vi "FilterHemisphereGPS.vi"(9 "Queue timeout (ms)":i32=200, 10 "NotifierReff":T2, 11 "Hemisphere Queue Cluster":T1) -> ()   [LabVIEW 2013]
doc: "Performs and filtering that we want (default is no filtering) and writes the data to the notifier. If no data is in the queue this VI times out after 'Queue timeout (ms)' has passed and nothing is written to the notifier.\n\nEric Schneider, March 2014"
uses:
  Data/TypeDefs/Notifiers.ctl
  Data/TypeDefs/UTM Location.ctl
  Data/TypeDefs/Sail Set Suggestions.ctl
  Data/TypeDefs/Rudder Set Suggestions.ctl
  Data/TypeDefs/OverrideInformation.ctl
  Data/TypeDefs/OverrideMode.ctl
  Data/TypeDefs/MotorSetup.ctl
  Data/TypeDefs/DynamixelSetupInfo.ctl
  Data/TypeDefs/AirmarStatus.ctl
  Data/TypeDefs/HardwareOnline.ctl
  Data/TypeDefs/DynamixelCycleTracker.ctl
  Data/TypeDefs/RC Input Values.ctl
  Classes/Waypoint/Waypoint.lvclass
  Data/TypeDefs/GPS-Compass Queue Cluster.ctl
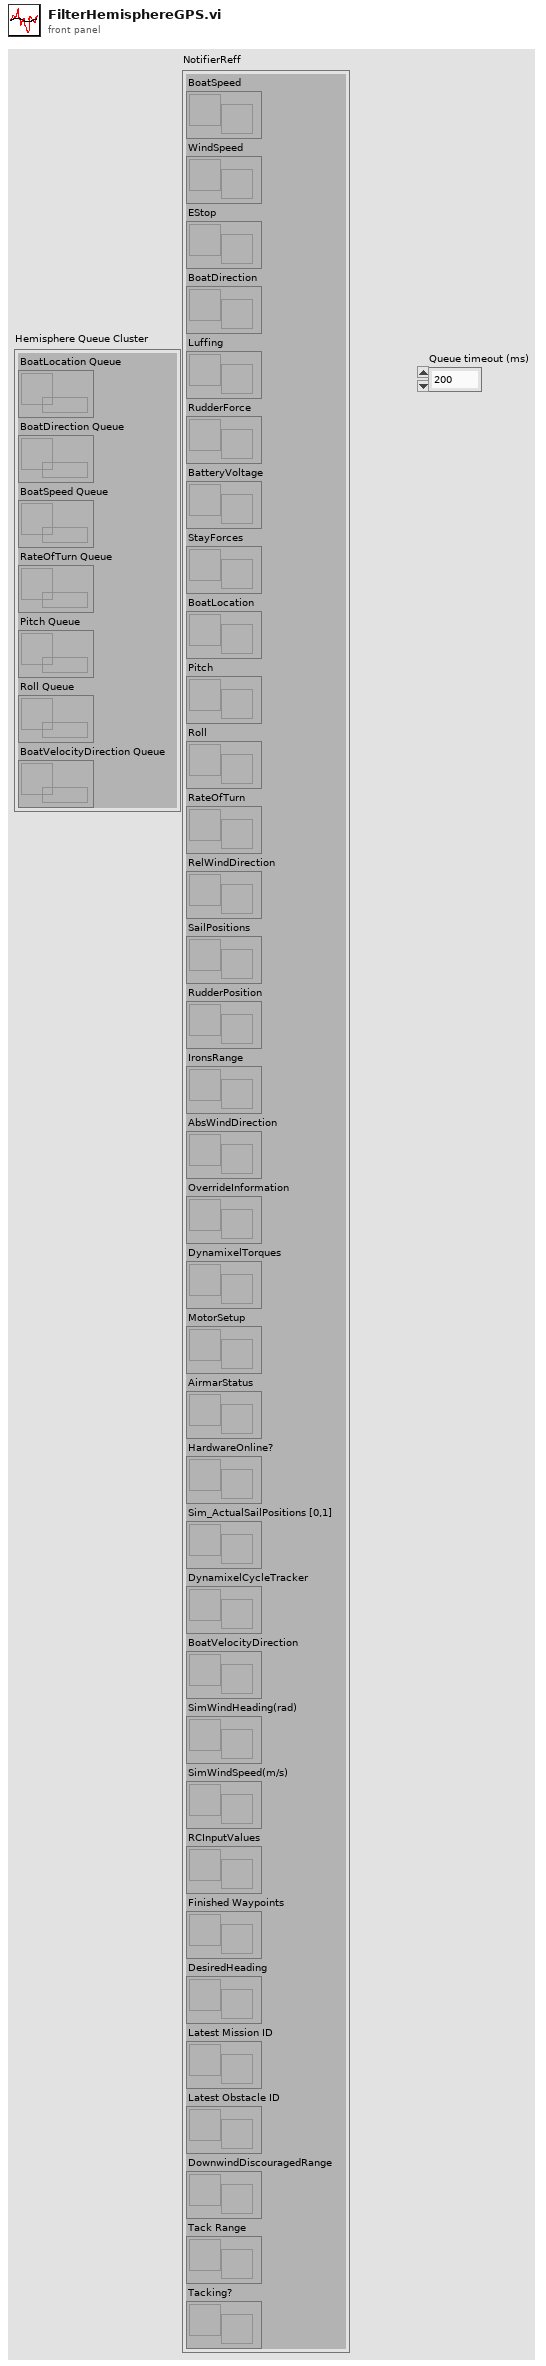
[diagram p1: front panel]
types:
  T1 = typedef "GPS-Compass Queue Cluster.ctl" = cluster{"BoatLocation Queue":refnum<queue>, "BoatDirection Queue":refnum<queue>, "BoatSpeed Queue":refnum<queue>, "RateOfTurn Queue":refnum<queue>, "Pitch Queue":refnum<queue>, "Roll Queue":refnum<queue>, "BoatVelocityDirection Queue ":refnum<queue>}
  T2 = typedef "Notifiers.ctl" = cluster{"BoatSpeed":refnum<notifier>, "WindSpeed":refnum<notifier>, "EStop":refnum<notifier>, "BoatDirection":refnum<notifier>, "Luffing":refnum<notifier>, "RudderForce":refnum<notifier>, "BatteryVoltage":refnum<notifier>, "StayForces":refnum<notifier>, "BoatLocation":refnum<notifier>, "Pitch":refnum<notifier>, "Roll":refnum<notifier>, "RateOfTurn":refnum<notifier>, "RelWindDirection":refnum<notifier>, "SailPositions":refnum<notifier>, "RudderPosition":refnum<notifier>, "IronsRange":refnum<notifier>, "AbsWindDirection":refnum<notifier>, "OverrideInformation":refnum<notifier>, "DynamixelTorques":refnum<notifier>, "MotorSetup":refnum<notifier>, "AirmarStatus":refnum<notifier>, "HardwareOnline?":refnum<notifier>, "Sim_ActualSailPositions [0,1]":refnum<notifier>, "DynamixelCycleTracker":refnum<notifier>, "BoatVelocityDirection":refnum<notifier>, "SimWindHeading(rad)":refnum<notifier>, "SimWindSpeed(m/s)":refnum<notifier>, "RCInputValues":refnum<notifier>, "Finished Waypoints":refnum<notifier>, "DesiredHeading":refnum<notifier>, "Latest Mission ID":refnum<notifier>, "Latest Obstacle ID":refnum<notifier>, "DownwindDiscouragedRange":refnum<notifier>, "Tack Range":refnum<notifier>, "Tacking?":refnum<notifier>}
  T3 = typedef "UTM Location.ctl" = cluster{"UTM Zone":dbl, "Hemisphere":enum16{"North", "South"}, "East":dbl, "North":dbl}
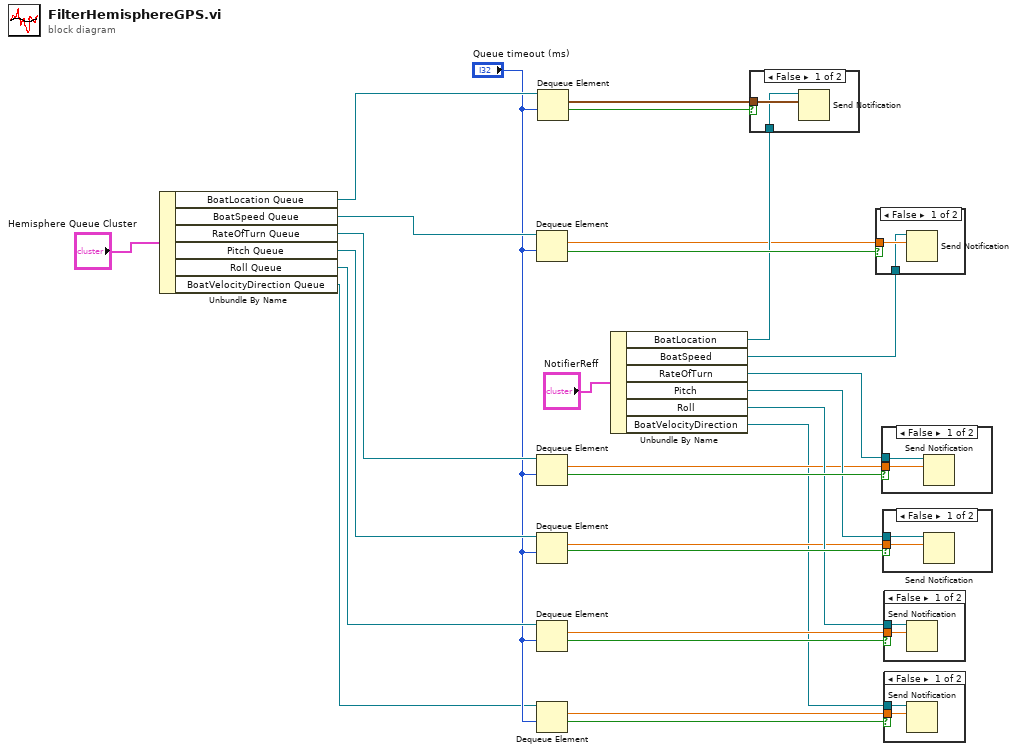
[diagram p0: block diagram]
diagram:
  n1 = Unbundle By Name("Hemisphere Queue Cluster") -> ("BoatLocation Queue"=w7:refnum<queue>, "BoatSpeed Queue"=w8:refnum<queue>, "RateOfTurn Queue"=w9:refnum<queue>, "Pitch Queue"=w10:refnum<queue>, "Roll Queue"=w11:refnum<queue>, "BoatVelocityDirection Queue"=w4:refnum<queue>)
  n2 = Dequeue Element(queue=w8, timeout in ms (-1)="Queue timeout (ms)") -> (element=w14:dbl, timed out?=w24:bool)  [unwired: 1 in, 2 out]
  n3 = Dequeue Element(queue=w9, timeout in ms (-1)="Queue timeout (ms)") -> (element=w13:dbl, timed out?=w25:bool)  [unwired: 1 in, 2 out]
  n4 = Dequeue Element(queue=w10, timeout in ms (-1)="Queue timeout (ms)") -> (element=w15:dbl, timed out?=w26:bool)  [unwired: 1 in, 2 out]
  n5 = Dequeue Element(queue=w11, timeout in ms (-1)="Queue timeout (ms)") -> (element=w16:dbl, timed out?=w27:bool)  [unwired: 1 in, 2 out]
  n6 = Dequeue Element(queue=w4, timeout in ms (-1)="Queue timeout (ms)") -> (element=w2:dbl, timed out?=w3:bool)  [unwired: 1 in, 2 out]
  n7 = Dequeue Element(queue=w7, timeout in ms (-1)="Queue timeout (ms)") -> (element=w12:T3, timed out?=w23:bool)  [unwired: 1 in, 2 out]
  n8 = Unbundle By Name("NotifierReff") -> ("BoatLocation"=w18:refnum<notifier>, "BoatSpeed"=w19:refnum<notifier>, "RateOfTurn"=w20:refnum<notifier>, "Pitch"=w21:refnum<notifier>, "Roll"=w22:refnum<notifier>, "BoatVelocityDirection"=w1:refnum<notifier>)
  n9 = case shown="False" w23 {
    tunnel: w12 -> [w29 _]
    tunnel: w18 -> [w28 _]
    frame False {
      n10 = Send Notification(notification=w29, notifier=w28) -> ()  [unwired: 1 in, 2 out]
    }
    frame True {
    }
  }
  n11 = case shown="False" w24 {
    tunnel: w14 -> [w31 _]
    tunnel: w19 -> [w30 _]
    frame False {
      n12 = Send Notification(notification=w31, notifier=w30) -> ()  [unwired: 1 in, 2 out]
    }
    frame True {
    }
  }
  n13 = case shown="False" w25 {
    tunnel: w13 -> [w33 _]
    tunnel: w20 -> [w32 _]
    frame False {
      n14 = Send Notification(notification=w33, notifier=w32) -> ()  [unwired: 1 in, 2 out]
    }
    frame True {
    }
  }
  n15 = case shown="False" w26 {
    tunnel: w15 -> [w35 _]
    tunnel: w21 -> [w34 _]
    frame False {
      n16 = Send Notification(notification=w35, notifier=w34) -> ()  [unwired: 1 in, 2 out]
    }
    frame True {
    }
  }
  n17 = case shown="False" w27 {
    tunnel: w16 -> [w37 _]
    tunnel: w22 -> [w36 _]
    frame False {
      n18 = Send Notification(notification=w37, notifier=w36) -> ()  [unwired: 1 in, 2 out]
    }
    frame True {
    }
  }
  n19 = case shown="False" w3 {
    tunnel: w2 -> [w39 _]
    tunnel: w1 -> [w38 _]
    frame False {
      n20 = Send Notification(notification=w39, notifier=w38) -> ()  [unwired: 1 in, 2 out]
    }
    frame True {
    }
  }
